vi "ClusterTestUI.vi"() -> ()   [LabVIEW 2016]
panel:
  in  "Text":string
  in  "Numeric":dbl
  in  "Cluster 9":T1
  in  "Tab Control":enum32{"Page 1", "Page 2"}(tab)
  in  "Cluster 5":T2
  in  "Cluster 6":T1
  in  "Tab Control 2":enum32{"Page 1", "Page 2"}(tab)
  in  "Cluster 7":T2
  in  "Cluster 8":T2
  in  "Cluster":T2
  in  "Cluster 2":T3
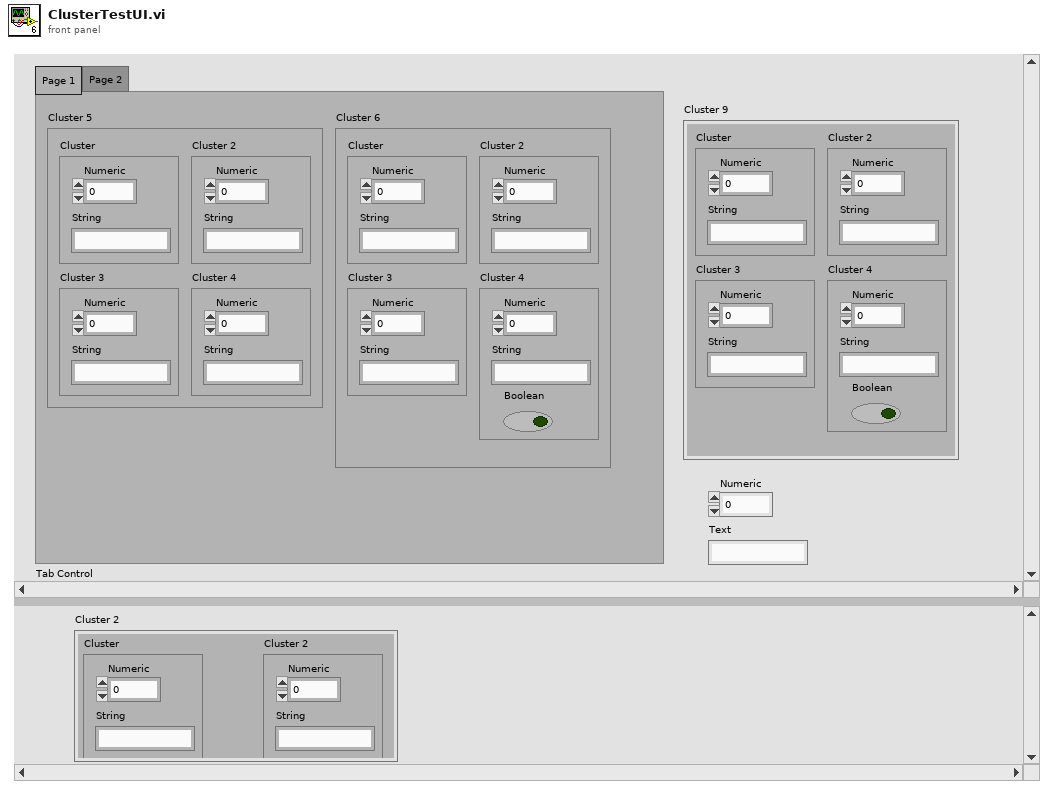
[diagram p1: front panel]
types:
  T1 = cluster{"Cluster":cluster{"Numeric":dbl, "String":string}, "Cluster 2":cluster{"Numeric":dbl, "String":string}, "Cluster 3":cluster{"Numeric":dbl, "String":string}, "Cluster 4":cluster{"Numeric":dbl, "String":string, "Boolean":bool}}
  T2 = cluster{"Cluster":cluster{"Numeric":dbl, "String":string}, "Cluster 2":cluster{"Numeric":dbl, "String":string}, "Cluster 3":cluster{"Numeric":dbl, "String":string}, "Cluster 4":cluster{"Numeric":dbl, "String":string}}
  T3 = cluster{"Cluster":cluster{"Numeric":dbl, "String":string}, "Cluster 2":cluster{"Numeric":dbl, "String":string}}
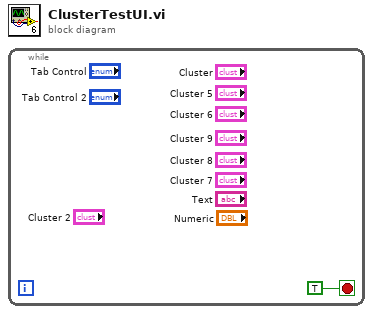
[diagram p0: block diagram]
diagram:
  n1 = while {
    stop <- TRUE stop-if-true
  }
